vi "data_headers_subVI_V2.vi"(8 "Experiment Notes":string, 10 "Sample names":T1={"QCM1 sample name"="aQCM2", "QCM2 sample name"="aQCM2", "QCM3 sample name"="aQCM3", "QCM4 sample name"="aQCM4", "QCM5 sample name"="aQCM5", "QCM6 sample name"="aQCM6", "SRS sample name"="sample_SRS", "Keithley 2420 sample name"="Keithley2420", "Keithley 6430 sample name"="Keithley6430", "Keithley 2100 sample name"="Keithley6430"}) -> (2 "data headers":string[](array[string]))   [LabVIEW 2014]
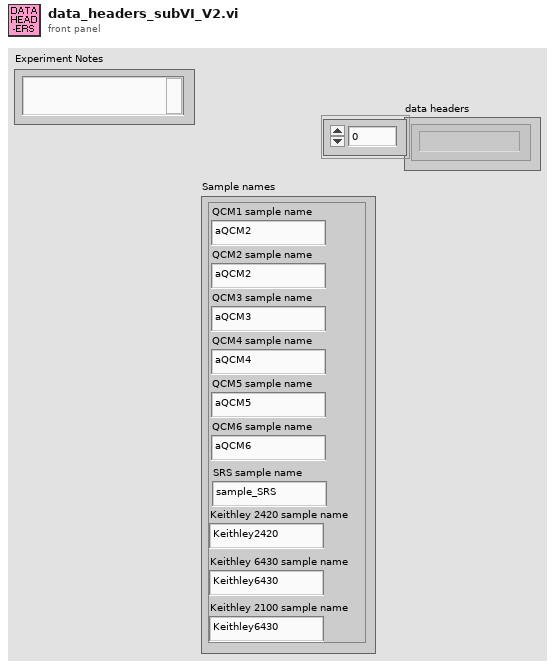
[diagram p1: front panel]
types:
  T1 = cluster{"QCM1 sample name":string, "QCM2 sample name":string, "QCM3 sample name":string, "QCM4 sample name":string, "QCM5 sample name":string, "QCM6 sample name":string, "SRS sample name":string, "Keithley 2420 sample name":string, "Keithley 6430 sample name":string, "Keithley 2100 sample name":string}
  T2 = cluster{string, string, string, string, string, string}
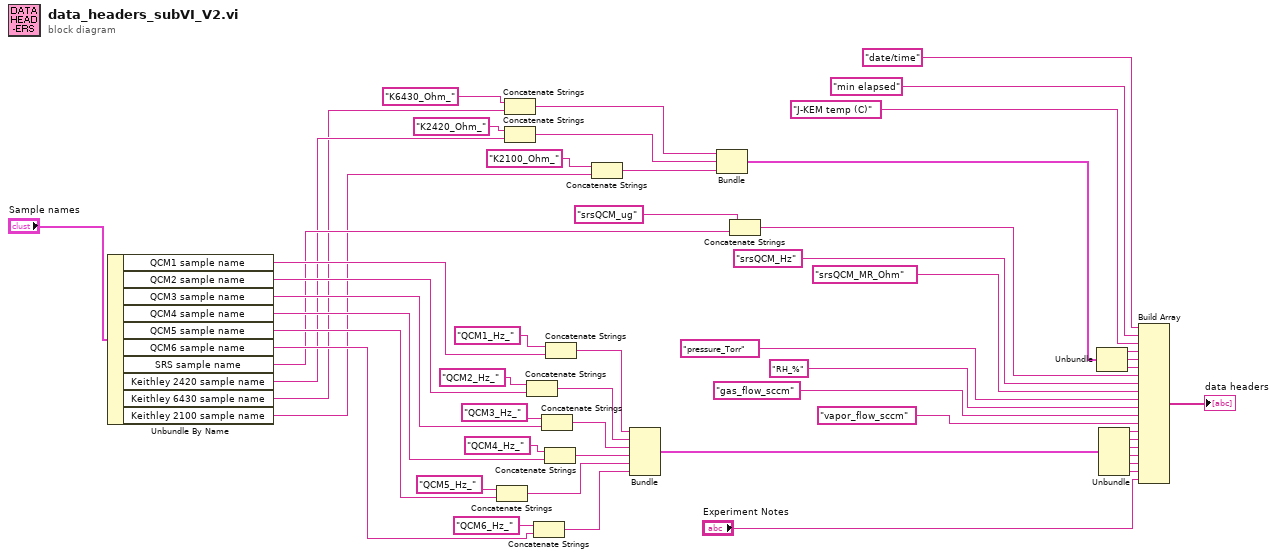
[diagram p0: block diagram]
diagram:
  n1 = Unbundle By Name("Sample names") -> ("QCM1 sample name"=w40:string, "QCM2 sample name"=w37:string, "QCM3 sample name"=w35:string, "QCM4 sample name"=w33:string, "QCM5 sample name"=w30:string, "QCM6 sample name"=w29:string, "SRS sample name"=w26:string, "Keithley 2420 sample name"=w25:string, "Keithley 6430 sample name"=w24:string, "Keithley 2100 sample name"=w22:string)
  n2 = Concatenate Strings("QCM5_Hz_" ("string"), w30) -> (w9:string)
  n3 = Concatenate Strings("K6430_Ohm_", w24) -> (w20:string)
  n4 = Concatenate Strings("K2420_Ohm_" ("element"), w25) -> (w19:string)
  n5 = Concatenate Strings("QCM2_Hz_" ("string"), w37) -> (w12:string)
  n6 = Concatenate Strings("QCM6_Hz_" ("string"), w29) -> (w8:string)
  n7 = Concatenate Strings("QCM3_Hz_" ("string"), w35) -> (w11:string)
  n8 = Concatenate Strings("QCM4_Hz_" ("string"), w33) -> (w10:string)
  n9 = Concatenate Strings("QCM1_Hz_" ("string"), w40) -> (w13:string)
  n10 = Concatenate Strings("K2100_Ohm_" ("element"), w22) -> (w18:string)
  n11 = Bundle(w13, w12, w11, w10, w9, w8) -> (w7:T2)  [unwired: 1 in]
  n12 = Bundle(w20, w19, w18) -> (w17:cluster{string, string, string})  [unwired: 1 in]
  n13 = Concatenate Strings("srsQCM_ug", w26) -> (w27:string)
  n14 = Unbundle(w17) -> (w16:string, w15:string, w14:string)
  n15 = Unbundle(w7) -> (w6:string, w5:string, w4:string, w3:string, w2:string, w1:string)
  n16 = Build Array("date/time", "min elapsed", "J-KEM temp (C)", w16, w15, w14, w27, "srsQCM_Hz", "srsQCM_MR_Ohm", "pressure_Torr" ("element"), "RH_%" ("element"), "gas_flow_sccm" ("element"), "vapor_flow_sccm" ("element"), w6, w5, w4, w3, w2, w1, "Experiment Notes") -> (→"data headers":string[])
